vi "Connect.vi"(8 "error in (no error)":errorcluster, 10 "URL":string, 11 "Network Actor in":refnum<class "Client LNA.lvclass">) -> (0 "error out":errorcluster, 3 "Network Actor out":refnum<class "Client LNA.lvclass">)   [LabVIEW 2026, in "Client LNA.lvlib" / "Client LNA.lvclass"]
doc: "Opens a connection to a remote Linked Network Actor reader stream, Sends a message to the remote Linked Network Actor to connect to the local reader stream."
uses:
  Client LNA.lvclass
  Client LNA.lvclass/Client LNA.ctl
  C:/Users/E2013170/Documents/GitHub/Measurement-Utility-Reference/recovery/packages/ni_lib_linked_network_actor-1.2.0.19-9492AF5A82/File Group 0/vi.lib/NI/Actors/Linked Network Actor/Linked Network Actor/Linked Network Actor.lvclass
  C:/Program Files/National Instruments/LabVIEW 2026/vi.lib/ActorFramework/Actor/Actor.lvclass
  C:/Users/E2013170/Documents/GitHub/Measurement-Utility-Reference/components/HAL-MAL-Application/Source/Framework/Client/Client LNA/Client LNA.lvclass
  <vilib>/ActorFramework/Actor/Actor.lvclass
  MAL-Framework/user.lib/Common Components/Controller/Messages/Log Status/Log Status.lvclass
  recovery/packages/ni_lib_linked_network_actor-1.2.0.19-9492AF5A82/File Group 0/vi.lib/NI/Actors/Linked Network Actor/Linked Network Actor/Linked Network Actor.lvclass
  Client Controller/Messages/LNA Connected Msg/LNA Connected Msg.lvclass
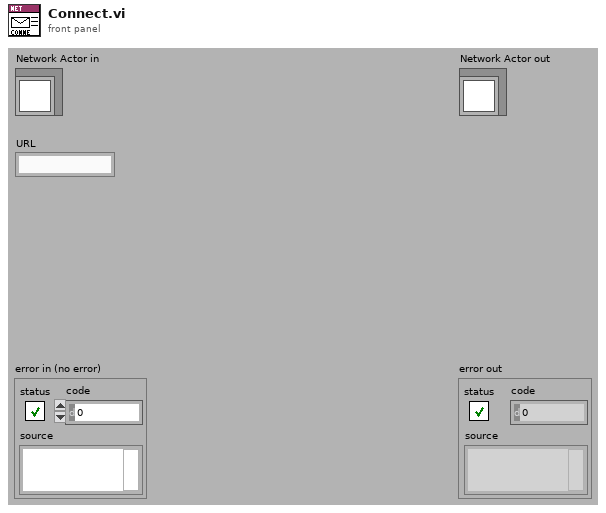
[diagram p1: front panel]
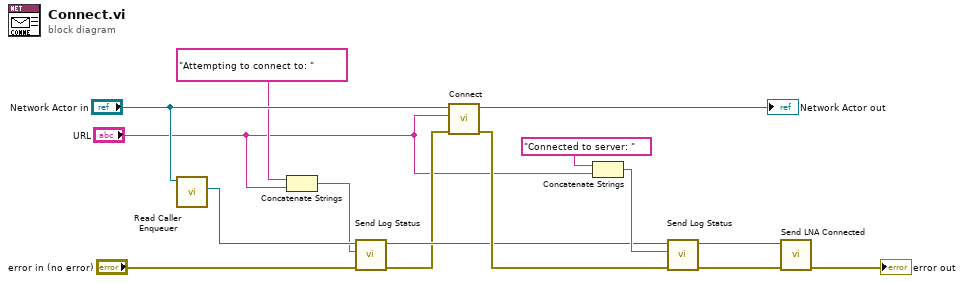
[diagram p0: block diagram]
diagram:
  n1 = call <vilib>:"Read Caller Enqueuer.vi"("Actor"="Network Actor in") -> ("Caller Enqueuer"=w10:refnum<class "Message Enqueuer.lvclass">)  [unwired: 10 in]
  n2 = Concatenate Strings("Attempting to connect to: " ("string"), "URL") -> (w4:string)
  n3 = call "Send Log Status.vi"("error in (no error)"="error in (no error)", "String"=w4, "Message Enqueuer in"=w10) -> ("error out"=w7:errorcluster, "Message Enqueuer out"=w9:refnum<class "Message Enqueuer.lvclass">)  [unwired: 7 in]
  n4 = call-parent "Connect.vi"("error in (no error)"=w7, "URL"="URL", "Network Actor in"="Network Actor in") -> ("error out"=w12:errorcluster, "Network Actor out"=→"Network Actor out":refnum<class "Client LNA.lvclass">)  [unwired: 7 in]
  n5 = Concatenate Strings("Connected to server: " ("string"), "URL") -> (w14:string)
  n6 = call "Send Log Status.vi"("error in (no error)"=w12, "String"=w14, "Message Enqueuer in"=w9) -> ("error out"=w3:errorcluster, "Message Enqueuer out"=w2:refnum<class "Message Enqueuer.lvclass">)  [unwired: 7 in]
  n7 = call "Send LNA Connected.vi"("error in (no error)"=w3, "Message Enqueuer"=w2) -> ("error out"=→"error out":errorcluster)  [unwired: 8 in, 1 out]
